vi "StartService.vi"(2 "LogPath in":path, 3 "New server ROS":T2) -> (0 "LogPath out":path, 1 "MyState":T1)   [LabVIEW 2015]
doc: "Starts a service and returns the state of the service"
uses:
  _ROSControl.ctl
  _ROSDirection.ctl
  Console/Servers/ServerSubs/MyState.ctl
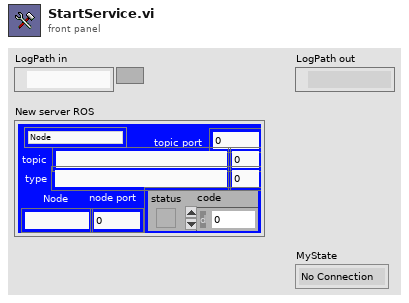
[diagram p1: front panel]
types:
  T1 = typedef "MyState.ctl" = enum16{"No Connection", "Registered", "Connected", "Close"}
  T2 = typedef "_ROSControl.ctl" = cluster{"topic port":u16, "Node":string, "topic":string, "type":string, "node port":u16, "error ":errorcluster, "Direction":T3, "Update (ms)":u16, "FIFO size":u16}
  T3 = typedef "_ROSDirection.ctl" = enum16{"Node", "Publisher", "Subscriber", "ServiceClient", "ServiceProvider"}
  T4 = enum16{"Reset Log", "Add Client", "Remove Client", "Add Task"}
  T5 = typedef "ROSLog.ctl" = cluster{"Sent":string, "Reply":string, "MethodName":string, "success":bool, "Dir1":string, "Dir2":string, "Time Stamp":string, "error":errorcluster, "Preamble":string, "Midamble":string, "Postamble":string}
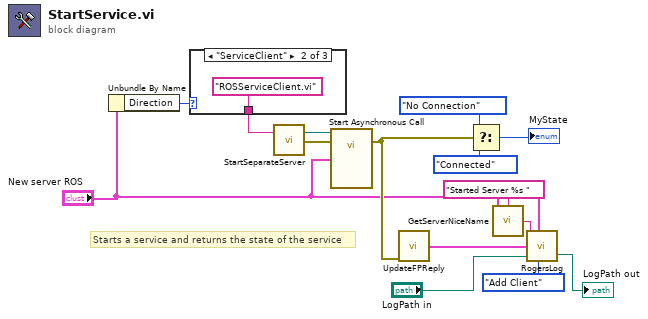
[diagram p0: block diagram]
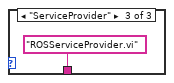
[diagram p3: hidden frame]
diagram:
  # "Starts a service and returns the state of the service"
  n1 = Unbundle By Name("New server ROS") -> ("Direction"=w1:T3)
  n2 = case shown="\"ServiceClient\"" w1 {
    tunnel: [_ "ROSServiceClient.vi" ("name (unnamed)") "ROSServiceProvider.vi" ("name (unnamed)")] -> w5
    frame Default {
    }
    frame "ServiceClient" {
    }
    frame "ServiceProvider" {
    }
  }
  n3 = call "StartSeparateServer.vi"("Server"=w5) -> ("error out"=w3:errorcluster, "Ref out"=w4:refnum<vi>)  [unwired: 1 in]
  n4 = call-by-ref "Start Asynchronous Call"(reference=w4, error in=w3, "ROS"="New server ROS") -> (error out=w9:errorcluster)  [unwired: 3 in, 1 out]
  n5 = call "UpdateFPReply.vi"("error in (no error)"=w9) -> ("Log"=w10:T5)  [unwired: 3 in]
  n6 = Select(t=MyState."No Connection" ("MyState"), s=w9, f=MyState."Connected" ("MyState")) -> (s? t:f=→"MyState":T1)
  n7 = call "GetServerNiceName.vi"("ROS"="New server ROS", "Text to add"="Started Server %s ") -> ("String"=w11:string)
  n8 = call "RogersLog.vi"("Text to add"=w11, "ROS"="New server ROS", "Log"=w10, "LogPath in"="LogPath in", "Task"=T4."Add Client") -> ("LogPath out"=→"LogPath out":path)  [unwired: 1 out]
